vi "Control_PID_System.vi"() -> ()   [LabVIEW 2021]
uses:
  <vilib>/Instr/_visa.llb/VISA Configure Serial Port (Instr).vi
  <vilib>/Utility/file.llb/Write Delimited Spreadsheet (DBL).vi
panel:
  out "ERRO":dbl(graph)
  out "Process Value":dbl format="%.1f"
  in  "Disturbance":dbl(slide)=10.0 min=10.0 max=20.0 step=0.10000000149011612 scale=10.0..20.0 scale format="%.1f"
  out "SYSTEM":cluster{dbl, "Process Value":dbl}(graph)
  out "CA":dbl
  out "SP":dbl
  out "D":dbl
  out "I":dbl
  out "P":dbl
  out "P,I,D,SP,CA,PV,e_rel(depois de passar pelo arduino)":string
  in  "Set Point(SP)":dbl(slide) scale=0.0..100.0
  in  "D":dbl
  in  "I":dbl
  in  "P":dbl
  in  "ON/OFF":bool
  in  "VISA resource name":refnum<visa-resource-name>
  # "VALORES NUMERICOS QUE SAEM DO ARDUINO\nPARA CONFIRMAR CORRETA RECE敲O DOS DADOS"
  # "INPUT:"
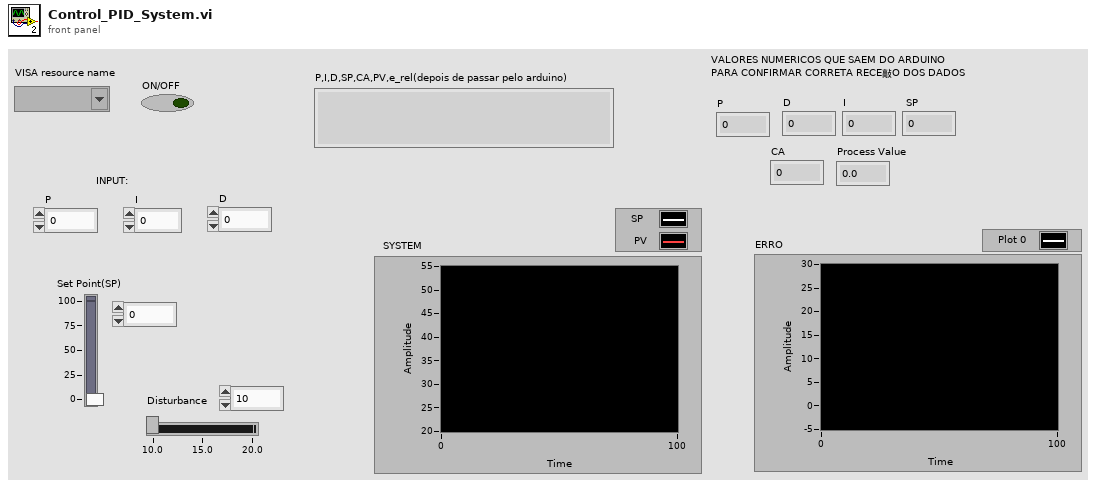
[diagram p1: front panel]
types:
  T1 = cluster{"Set Point(SP)":dbl, "Process Value":dbl}
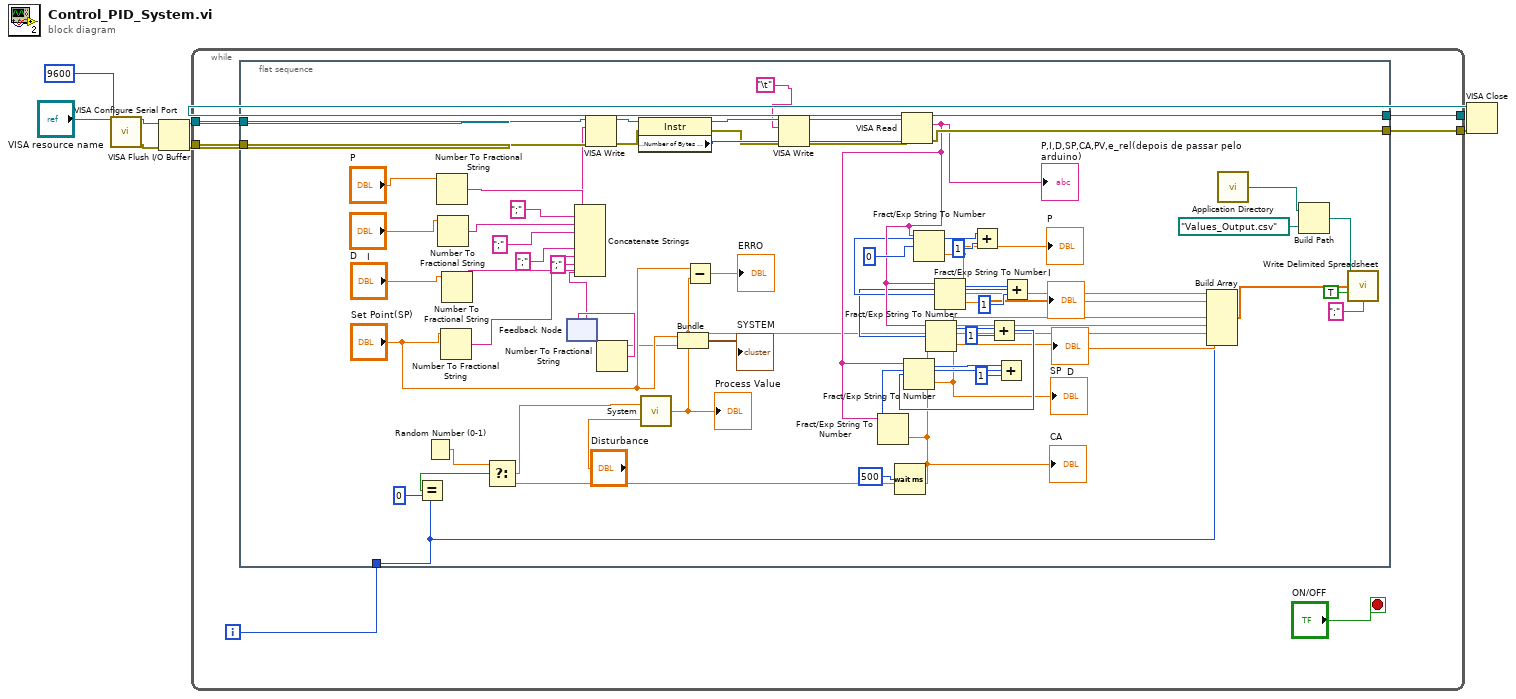
[diagram p0: block diagram]
diagram:
  n1 = call-poly "VISA Configure Serial Port"("VISA resource name"="VISA resource name", "baud rate (9600)"=u32 9600) -> ("VISA resource name out"=w2:refnum<visa-resource-name>, "error out"=w1:errorcluster)  [unwired: 12 in]
  n2 = VISA Flush I/O Buffer(VISA resource name=w2, error in (no error)=w1) -> (VISA resource name out=w4:refnum<visa-resource-name>, error out=w3:errorcluster)  [unwired: 1 in]
  n3 = while {
    tunnel: w4 -> [w13]
    tunnel: w3 -> [w12]
    tunnel: [w11] -> w6
    tunnel: [w10] -> w5
    i -> [w9]
    stop <- "ON/OFF" stop-if-true
    n4 = flat-sequence {
      tunnel: [w76] -> w11
      tunnel: [w75] -> w10
      tunnel: w13 -> [w51]
      tunnel: w12 -> [w50]
      tunnel: w9 -> [w18]
      frame #0 {
        n5 = Equal?(x=w18, y=0) -> (x = y?=w35:bool)
        n6 = Random Number (0-1)() -> (number: 0 to 1=w34:dbl)
        n7 = Number To Fractional String(number="P") -> (F-format string=w44:string)  [unwired: 3 in]
        n8 = Number To Fractional String(number="I") -> (F-format string=w42:string)  [unwired: 3 in]
        n9 = Number To Fractional String(number="Set Point(SP)") -> (F-format string=w38:string)  [unwired: 3 in]
        n10 = Number To Fractional String(number="D") -> (F-format string=w40:string)  [unwired: 3 in]
        n11 = feedback #1() -> (w30:string)  [unwired: 1 in]
        n12 = Concatenate Strings(w44, ";" ("string"), w42, ";" ("string"), w40, ";" ("string"), w38, ";" ("string"), w30) -> (w37:string)
        n13 = VISA Write(VISA resource name=w51, write buffer=w37, error in (no error)=w50) -> (VISA resource name out=w49:refnum<visa-resource-name>, error out=w48:errorcluster)  [unwired: 1 out]
        n14 = property class="Instr"(reference=w49, error in=w48) -> (reference out=w54:refnum<visa-resource-name>, error out=w53:errorcluster, "Serial Settings:Number of Bytes at Serial Port"=w71:u32)
        n15 = VISA Write(VISA resource name=w54, write buffer="\t", error in (no error)=w53) -> (VISA resource name out=w73:refnum<visa-resource-name>, error out=w72:errorcluster)  [unwired: 1 out]
        n16 = Wait (ms)(milliseconds to wait=u32 500) -> ()  [unwired: 1 out]
        n17 = VISA Read(VISA resource name=w73, byte count=w71, error in (no error)=w72) -> (VISA resource name out=w76:refnum<visa-resource-name>, read buffer=w69:string, error out=w75:errorcluster)  [unwired: 1 out]
        "P,I,D,SP,CA,PV,e_rel(depois de passar pelo arduino)" <- w69
        n18 = Fract/Exp String To Number(string=w69, offset=0) -> (offset past number=w66:i32, number=w26:dbl)  [unwired: 2 in]
        "P" <- w26
        n19 = Add(x=w66, y=1) -> (x+y=w63:i32)
        n20 = Fract/Exp String To Number(string=w69, offset=w63) -> (offset past number=w64:i32, number=w25:dbl)  [unwired: 2 in]
        "I" <- w25
        n21 = Add(x=w64, y=1) -> (x+y=w61:i32)
        n22 = Fract/Exp String To Number(string=w69, offset=w61) -> (offset past number=w60:i32, number=w24:dbl)  [unwired: 2 in]
        "D" <- w24
        n23 = Add(x=w60, y=1) -> (x+y=w58:i32)
        n24 = Fract/Exp String To Number(string=w69, offset=w58) -> (offset past number=w57:i32, number=w23:dbl)  [unwired: 2 in]
        "SP" <- w23
        n25 = Add(x=w57, y=1) -> (x+y=w55:i32)
        n26 = Fract/Exp String To Number(string=w69, offset=w55) -> (number=w22:dbl)  [unwired: 2 in, 1 out]
        "CA" <- w22
        n27 = Select(t=w34, s=w35, f=w22) -> (s? t:f=w33:dbl)
        n28 = call "System.vi"("Disturbance"="Disturbance", "Control Action"=w33) -> ("Process Value"=w16:dbl)
        "Process Value" <- w16
        n29 = Number To Fractional String(number=w16) -> (F-format string=w31:string)  [unwired: 3 in]
        n30 = feedback-in #1(w31) -> ()
        n31 = Bundle("Set Point(SP)"="Set Point(SP)", "Process Value"=w16) -> (→"SYSTEM":T1)  [unwired: 1 in]
        n32 = Subtract(x="Set Point(SP)", y=w16) -> (x-y=→"ERRO":dbl)
        n33 = Build Array(w26, w25, w24, w23, w22, w16, w18) -> (w21:dbl[])
        n34 = call <vilib>:"Application Directory.vi"() -> ("Application Directory"=w29:path)
        n35 = Build Path(base path=w29, name or relative path=path "Values_Output.csv") -> (appended path=w27:path)
        n36 = call-poly <vilib>:"Write Delimited Spreadsheet.vi"("file path (dialog if empty)"=w27, "1D data"=w21, "append to file? (new file:F)"=TRUE, "delimiter (\\t)"=";" ("delimiter (\\t)")) -> ()  [unwired: 10 in, 2 out]
      }
    }
  }
  n37 = VISA Close(VISA resource name=w6, error in (no error)=w5) -> ()  [unwired: 1 out]
